vi "Renishaw-XL80_GetHumidity.vi"(8 "error in (no error)":errorcluster, 11 "Renishaw-XL80 in":refnum<class "Renishaw-XL80.lvclass">) -> (0 "error out":errorcluster, 1 "pStatus":i32(ring) items=["SENSOR_OK"=0, "SENSOR_BAD_READING"=1, "SENSOR_FAILED"=2, "SENSOR_NOT_CONNECTED"=4], 2 "GetHumidity":dbl, 3 "Renishaw-XL80 out":refnum<class "Renishaw-XL80.lvclass">)   [LabVIEW 2024, in "Renishaw-XL80.lvclass"]
doc: "This method gets the latest reading (in %RH) and status from the air humidity sensor.\n\nDefinition\nHRESULTGetHumidity( [out] SENSOR_STATUS_CODES *pStatus, [out, retval] double *pVal);\nParameters\npStatus\nA variable that will be set to one of the SENSOR_STATUS_CODES.\n\npVal\nA variable that will be set to the air humidity reading (in %RH).\n\nComments\nIf the client has not connected to the DX10 then the default value (50 %RH) will be returned and the status will be set to SENSOR_NOT_CONNECTED.\n\nIf the client connected to a DX10 and it subsequently stopped responding, or the EC10 stopped responding then the last values obtained from the EC10 will be returned i.e. the status will not be modified. It is important therefore to monitor both the DX10Status and EC10Status. This is easily done using the _RenishawDX10Events interface.\n\nIf the sensor status is SENSOR_NOT_CONNECTED or SENSOR_BAD_READING, then pVal will be set to the last known valid reading.\n\nThe property will normally return an HRESULT of S_OK. However, it will return E_POINTER if the client supplies a null pointer for either pVal or pStatus.\n\nSee"
uses:
  Renishaw-XL80.lvclass
  Renishaw-XL80.lvclass/Renishaw-XL80.ctl
  D:/A.C.M/Example CSharp_64/bin/Debug/Interop.DX10SDKADAPTORLib.dll
  Example CSharp_64/bin/Debug/Interop.DX10SDKADAPTORLib.dll
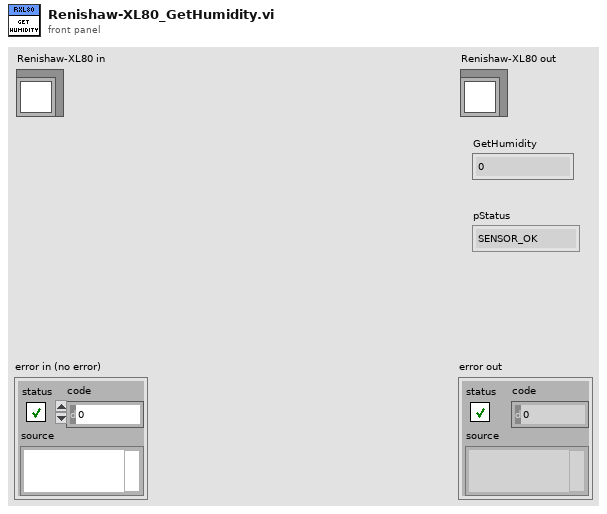
[diagram p1: front panel]
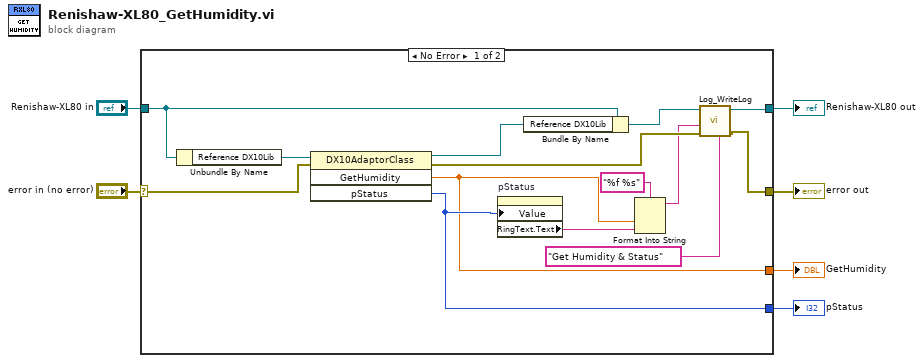
[diagram p0: block diagram]
diagram:
  n1 = case shown="No Error" "error in (no error)" {
    selector: "error in (no error)" -> [w14 w22]
    tunnel: [w13 w22] -> w5
    tunnel: [w16 w21] -> w3
    tunnel: "Renishaw-XL80 in" -> [w18 w21]
    tunnel: [w12 _] -> w2
    tunnel: [w10 _] -> w1
    frame No Error {
      n2 = Unbundle By Name(w18) -> ("Reference DX10Lib"=w19:refnum<k24>)
      n3 = invoke class="DX10AdaptorClass" method="GetHumidity"(reference=w19, error in=w14) -> (reference out=w20:refnum<k24>, error out=w15:errorcluster, "GetHumidity"=w10:dbl, "pStatus"=w12:i32)  [unwired: 2 in]
      n4 = property on="pStatus" class="Ring (strict)"("Value"=w12) -> ("RingText.Text"=w9:string)  [unwired: 2 in, 2 out]
      n5 = Bundle By Name(cluster=w18, "Reference DX10Lib"=w20) -> (w17:refnum<class "Renishaw-XL80.lvclass">)
      n6 = Format Into String(format string="%f %s", w10, w9) -> (resulting string=w8:string)  [unwired: 2 in, 1 out]
      n7 = call-dynamic "Log_WriteLog.vi"("Additional text"="Get Humidity & Status", "error in (no error)"=w15, "Response"=w8, "Log in"=w17) -> ("error out"=w13:errorcluster, "Log out"=w16:refnum<class "Renishaw-XL80.lvclass">)  [unwired: 6 in]
    }
    frame Error {
    }
  }
  "error out" <- w5
  "Renishaw-XL80 out" <- w3
  "pStatus" <- w2
  "GetHumidity" <- w1
